vi "Initialize.vi"(8 "error in (no error)":errorcluster, 9 "Data Cluster (for Headers)":variant, 10 "TableLogger Config":T1, 11 "object in":refnum<class "TableLogger_CSV_Actor.lvclass">) -> (0 "error out":errorcluster, 3 "object out":refnum<class "TableLogger_CSV_Actor.lvclass">)   [LabVIEW 2015, in "TableLogger_CSV_Actor.lvlib" / "TableLogger_CSV_Actor.lvclass"]
uses:
  TableLogger_CSV_Actor.lvclass
  TableLogger_Actor/TableLoggerConfig.ctl
  TableLogger_Actor/TableLoggerTypes.ctl
  TableLogger_CSV_Actor.lvclass/TableLogger_CSV_Actor.ctl
  <userlib>/_OpenG.lib/file/file.llb/File Exists - Scalar__ogtk.vi
  <userlib>/_OpenG.lib/file/file.llb/Build Path - Traditional__ogtk.vi
  LVdataToTableData/LVdataToTableData.lvlib
  TableLogger_Actor/TableLogger_Actor.lvlib
panel:
  # "Connector Pane"
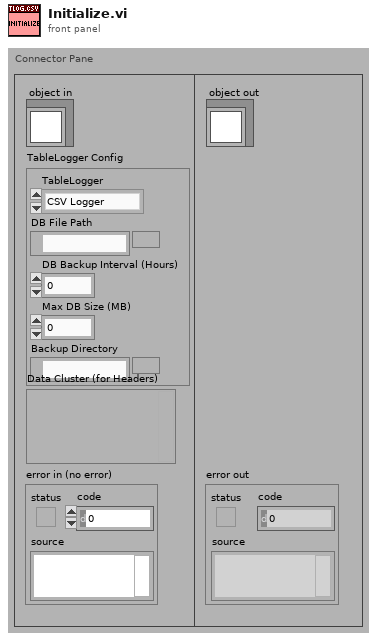
[diagram p1: front panel]
types:
  T1 = typedef "TableLogger_Actor.lvlib/TableLoggerConfig.ctl" = cluster{"TableLogger":T2, "DB File Path":path, "DB Backup Interval (Hours)":i32, "Max DB Size (MB)":i32, "Backup Directory":path}
  T2 = typedef "TableLogger_Actor.lvlib/TableLoggerTypes.ctl" = enum16{"CSV Logger", "SQLite Logger"}
  T3 = enum16{"open", "replace", "create", "open or create", "replace or create", "replace or create with confirmation"}
  T4 = typedef "Type Descriptor Enumeration__ogtk.ctl" = enum8{"<Null>", "I8", "I16", "I32", "I64", "U8", "U16", "U32", "U64", "SGL", "DBL", "EXT", "CSG", "CDB", "CXT", "0x0F", "0x10", "0x11", "0x12", "0x13", "0x14", "Enum U8", "Enum U16", "Enum U32", "Enum U64", "SGL PQ", "DBL PQ", "EXT PQ", "CSG PQ", "CDB PQ", "CXT PQ", "0x1F", "0x20", "Boolean", "0x22", "0x23", "0x24", "0x25", "0x26", "0x27", "0x28", "0x29", "0x2A", "0x2B", "0x2C", "0x2D", "0x2E", "0x2F", "String", "0x31", "Path", "Pict", "0x34", "0x35", "0x36", "DAQ", "0x38", "0x39", "0x3A", "0x3B", "0x3C", "0x3D", "0x3E", "0x3F", "Array", "0x41", "0x42", "0x43", "0x44", "0x45", "0x46", "0x47", "0x48", "0x49", "0x4A", "0x4B", "0x4C", "0x4D", "0x4E", "0x4F", "Cluster", "0x51", "0x52", "Variant", "Waveform", "0x55", "0x56", "0x57", "0x58", "0x59", "0x5A", "0x5B", "0x5C", "0x5D", "0x5E", "0x5F", "0x60", "0x61", "0x62", "0x63", "0x64", "0x65", "0x66", "0x67", "0x68", "0x69", "0x6A", "0x6B", "0x6C", "0x6D", "0x6E", "0x6F", "Refnum"}
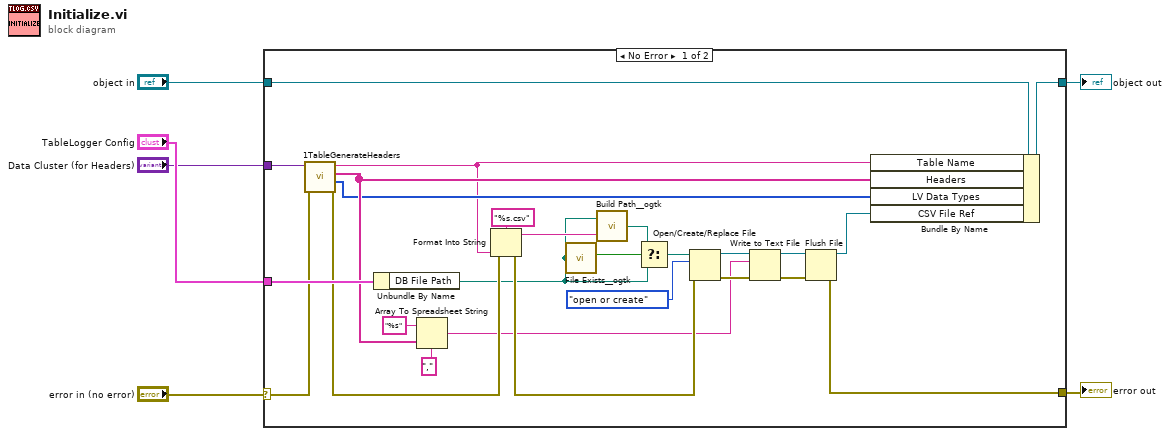
[diagram p0: block diagram]
diagram:
  n1 = case shown="No Error" "error in (no error)" {
    selector: "error in (no error)" -> [w24 w34]
    tunnel: [w14 w34] -> w6
    tunnel: [w23 w33] -> w5
    tunnel: "object in" -> [w32 w33]
    tunnel: "Data Cluster (for Headers)" -> [w31 _]
    tunnel: "TableLogger Config" -> [w29 _]
    frame No Error {
      n2 = call "1TableGenerateHeaders.vi"("error in (no error)"=w24, "Cluster Variant"=w31) -> ("error out"=w25:errorcluster, "LV Data Types"=w10:T4[], "Headers"=w11:string[], "Table Name"=w9:string)  [unwired: 6 in]
      n3 = Unbundle By Name(w29) -> ("DB File Path"=w7:path)
      n4 = Array To Spreadsheet String(delimiter (Tab)="," ("delimiter (\\t)"), array=w11, 3:"%s" ("format string")) -> (spreadsheet string=w16:string)
      n5 = Format Into String(format string="%s.csv", error in=w25, w9) -> (resulting string=w28:string, error out=w19:errorcluster)  [unwired: 1 in]
      n6 = call-poly <userlib>:"File Exists__ogtk.vi"("file path"=w7) -> ("is directory"=w30:bool)  [unwired: 6 in, 1 out]
      n7 = call-poly <userlib>:"Build Path__ogtk.vi"("name or relative path"=w28, "base path"=w7) -> ("appended path"=w26:path)
      n8 = Select(t=w26, s=w30, f=w7) -> (s? t:f=w22:path)
      n9 = Open/Create/Replace File(file path (use dialog)=w22, error in=w19, operation (0:open)=T3."open or create") -> (refnum out=w17:refnum<file>, error out=w18:errorcluster)  [unwired: 3 in, 1 out]
      n10 = Write to Text File(file (use dialog)=w17, text=w16, error in=w18) -> (refnum out=w13:refnum<file>, error out=w15:errorcluster)  [unwired: 1 in, 1 out]
      n11 = Flush File(refnum=w13, error in=w15) -> (refnum out=w12:refnum<file>, error out=w14:errorcluster)
      n12 = Bundle By Name(cluster=w32, "Table Name"=w9, "Headers"=w11, "LV Data Types"=w10, "CSV File Ref"=w12) -> (w23:refnum<class "TableLogger_CSV_Actor.lvclass">)
    }
    frame Error {
    }
  }
  "error out" <- w6
  "object out" <- w5
